vi "Read-Temp.vi"(7 "Slave Address (7-bit)":u8 format="%x", 8 "error in (no error)":errorcluster, 10 "Comp Coeffs":T1 {"dig_H6" format="%0d"; "dig_H5" format="%0d"; "dig_H4" format="%0d"; "dig_H3" format="%0d"; "dig_H2" format="%0d"; "dig_H1" format="%0d"; "dig_P9" format="%0d"; "dig_P8" format="%0d"; "dig_P7" format="%0d"; "dig_P6" format="%0d"; "dig_P5" format="%0d"; "dig_P4" format="%0d"; "dig_P3" format="%0d"; "dig_P2" format="%0d"; "dig_P1" format="%0d"; "dig_T3" format="%0d"; "dig_T2" format="%0d"; "dig_T1" format="%0d"}, 11 "I2C Ref Out in":T2) -> (0 "error out":errorcluster, 1 "T_fine":dbl format="%.2f", 2 "Comp Coeffs Out":T1 {"dig_H6" format="%0d"; "dig_H5" format="%0d"; "dig_H4" format="%0d"; "dig_H3" format="%0d"; "dig_H2" format="%0d"; "dig_H1" format="%0d"; "dig_P9" format="%0d"; "dig_P8" format="%0d"; "dig_P7" format="%0d"; "dig_P6" format="%0d"; "dig_P5" format="%0d"; "dig_P4" format="%0d"; "dig_P3" format="%0d"; "dig_P2" format="%0d"; "dig_P1" format="%0d"; "dig_T3" format="%0d"; "dig_T2" format="%0d"; "dig_T1" format="%0d"}, 3 "I2C Ref Out out":T2, 4 "ADC RAW TEMP":i32, 5 "Bytes Read Temp":u8[](array[numeric]), 6 "T":dbl)   [LabVIEW 2015]
uses:
  <vilib>/myRIO/Instrument Drivers/Onboard IO/I2C/typedefs/I2C Reference.ctl
  <vilib>/myRIO/Common/Instrument Driver Framework/Utilities/typedefs/myRIO Generic Hardware Reference.ctl
  <vilib>/myRIO/Common/Instrument Driver Framework/Utilities/typedefs/Hardware Version Enum.ctl
  <vilib>/myRIO/Common/Instrument Driver Framework/Utilities/typedefs/myRIO v1.0 Reference.ctl
  <vilib>/myRIO/Common/Instrument Driver Framework/Utilities/typedefs/Generic FPGA Reference.ctl
  <vilib>/myRIO/Common/Instrument Driver Framework/myRIO v1.0/I2C/typedefs/I2C Channels Enum.ctl
  <vilib>/myRIO/Instrument Drivers/Onboard IO/I2C/typedefs/I2C Configuration.ctl
  <vilib>/myRIO/Instrument Drivers/Onboard IO/I2C/typedefs/I2C Transfer Rate.ctl
  calib_data.ctl
  <vilib>/Utility/error.llb/Error Cluster From Error Code.vi
  <vilib>/myRIO/Common/Instrument Driver Framework/myRIO v1.0/I2C/vis/myRIO v1.0 Write I2C.vi
  <vilib>/myRIO/Common/Instrument Driver Framework/myRIO v1.0/I2C/vis/myRIO v1.0 Read I2C.vi
  <vilib>/myRIO/Instrument Drivers/Onboard IO/I2C/I2C.lvlib
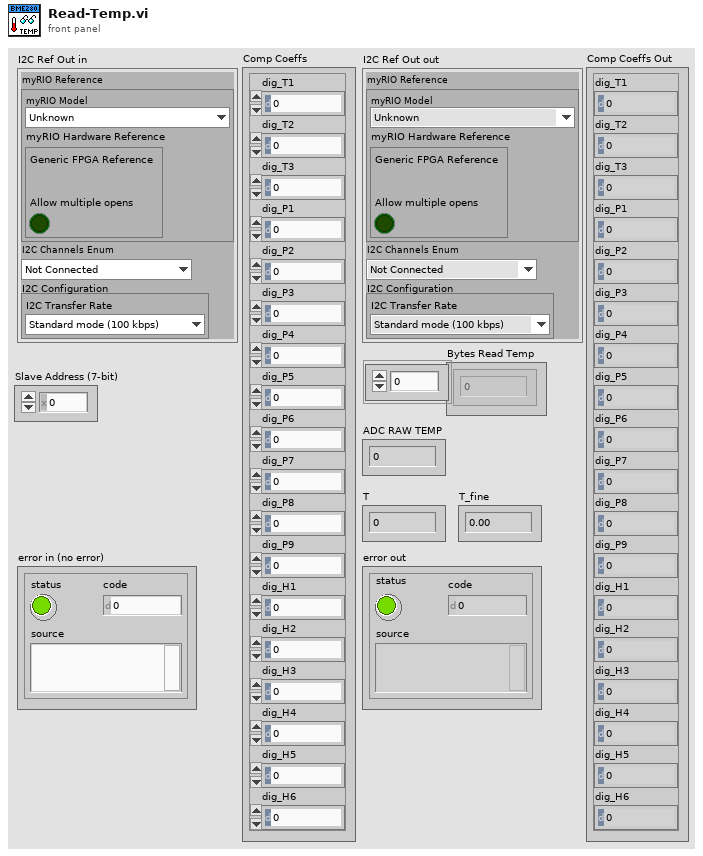
[diagram p1: front panel]
types:
  T1 = typedef "calib_data.ctl" = cluster{"dig_T1":u16, "dig_T2":i16, "dig_T3":i16, "dig_P1":u16, "dig_P2":i16, "dig_P3":i16, "dig_P4":i16, "dig_P5":i16, "dig_P6":i16, "dig_P7":i16, "dig_P8":i16, "dig_P9":i16, "dig_H1":u8, "dig_H2":i16, "dig_H3":u8, "dig_H4":i16, "dig_H5":i16, "dig_H6":i8}
  T2 = typedef "I2C.lvlib/I2C Reference.ctl" = cluster{"myRIO Reference":T3, "I2C Channels Enum":T7, "I2C Configuration":T8}
  T3 = typedef "myRIO Generic Hardware Reference.ctl" = cluster{"myRIO Model":T4, "myRIO Hardware Reference":T5}
  T4 = typedef "Hardware Version Enum.ctl" = enum16{"Unknown", "myRIO-1900", "myRIO-1950", "roboRIO"}
  T5 = typedef "myRIO v1.0 Reference.ctl" = cluster{"Generic FPGA Reference":T6, "Allow multiple opens":bool}
  T6 = typedef "Generic FPGA Reference.ctl" = refnum<k20>
  T7 = typedef "I2C Channels Enum.ctl" = enum16{"Not Connected", "A/I2C", "B/I2C", "I2C/I2C"}
  T8 = typedef "I2C.lvlib/I2C Configuration.ctl" = cluster{"I2C Transfer Rate":T9}
  T9 = typedef "I2C.lvlib/I2C Transfer Rate.ctl" = enum16{"Standard mode (100 kbps)", "Fast mode (400 kbps)"}
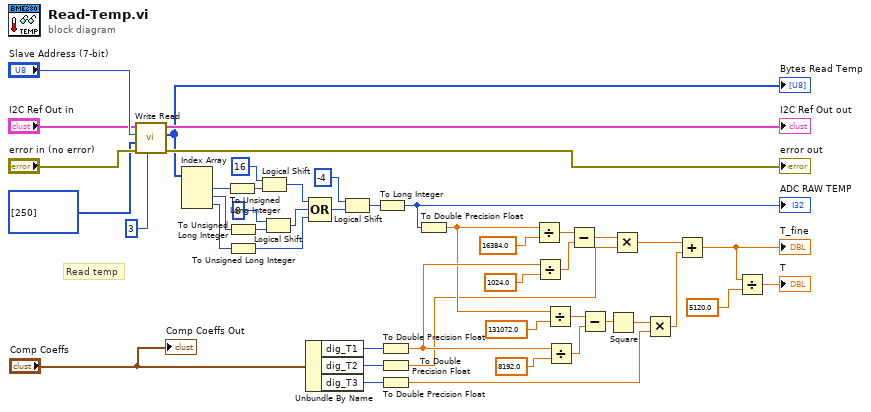
[diagram p0: block diagram]
diagram:
  # "Read temp"
  n1 = call <vilib>:"Write Read.vi"("Byte Count"=u32 3, "error in (no error)"="error in (no error)", "Bytes to Write"=u8[] [250], "Slave Address (7-bit)"="Slave Address (7-bit)", "I2C Ref In"="I2C Ref Out in") -> ("error out"=→"error out":errorcluster, "Bytes Read"=w8:u8[], "I2C Ref Out"=→"I2C Ref Out out":T2)  [unwired: 3 in]
  "Bytes Read Temp" <- w8
  n2 = Index Array(array=w8) -> (element #1=w9:u8, element #2=w10:u8, element #3=w11:u8)  [unwired: 3 in]
  n3 = To Unsigned Long Integer(number=w9) -> (unsigned 32bit integer=w17:u32)
  n4 = To Unsigned Long Integer(number=w10) -> (unsigned 32bit integer=w18:u32)
  n5 = To Unsigned Long Integer(number=w11) -> (unsigned 32bit integer=w13:u32)
  n6 = Logical Shift(y=u8 16 ("x"), x=w17) -> (x << y=w12:u32)
  n7 = Logical Shift(y=u8 8 ("x"), x=w18) -> (x << y=w14:u32)
  n8 = Unbundle By Name("Comp Coeffs") -> ("dig_T1"=w3:u16, "dig_T2"=w2:i16, "dig_T3"=w1:i16)
  n9 = Compound Arithmetic op=OR(w12, w14, w13) -> (w19:u32)
  n10 = Logical Shift(y=i16 -4, x=w19) -> (x << y=w23:u32)
  n11 = To Long Integer(number=w23) -> (32bit integer=w4:i32)
  "ADC RAW TEMP" <- w4
  n12 = To Double Precision Float(number=w3) -> (double precision float=w38:dbl)
  n13 = To Double Precision Float(number=w2) -> (double precision float=w32:dbl)
  n14 = To Double Precision Float(number=w1) -> (double precision float=w41:dbl)
  n15 = To Double Precision Float(number=w4) -> (double precision float=w37:dbl)
  n16 = Divide(x=w37, y=16384.0) -> (x/y=w29:dbl)
  n17 = Divide(x=w38, y=1024.0) -> (x/y=w30:dbl)
  n18 = Divide(x=w37, y=131072.0) -> (x/y=w34:dbl)
  n19 = Divide(x=w38, y=8192.0) -> (x/y=w33:dbl)
  n20 = Subtract(x=w29, y=w30) -> (x-y=w31:dbl)
  n21 = Subtract(x=w34, y=w33) -> (x-y=w39:dbl)
  n22 = Square(x=w39) -> (x^2=w40:dbl)
  n23 = Multiply(x=w31, y=w32) -> (x*y=w42:dbl)
  n24 = Multiply(x=w40, y=w41) -> (x*y=w43:dbl)
  n25 = Add(x=w42, y=w43) -> (x+y=w5:dbl)
  "T_fine" <- w5
  n26 = Divide(x=w5, y=5120.0) -> (x/y=→"T":dbl)
  "Comp Coeffs Out" <- "Comp Coeffs"
